vi "Get Topic.vi"(8 "error in (no error)":errorcluster, 9 "Topic Type":variant, 10 "Topic Name":string, 11 "TopicLookupTable in":refnum<class "TopicLookupTable.lvclass">) -> (0 "error out":errorcluster, 1 "Topic Found?":bool, 2 "Topic Refnum":refnum<class "Message Enqueuer.lvclass">, 3 "TopicLookupTable out":refnum<class "TopicLookupTable.lvclass">)   [LabVIEW 2015, in "Mediator.lvlib" / "TopicLookupTable.lvclass"]
uses:
  TopicLookupTable.lvclass
  <vilib>/ActorFramework/Message Enqueuer/Message Enqueuer.lvclass
  TopicLookupTable.lvclass/TopicLookupTable.ctl
  Topic/Topic.lvclass
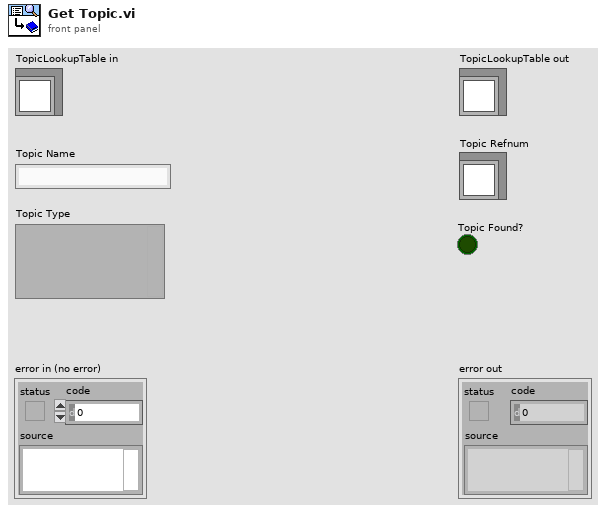
[diagram p1: front panel]
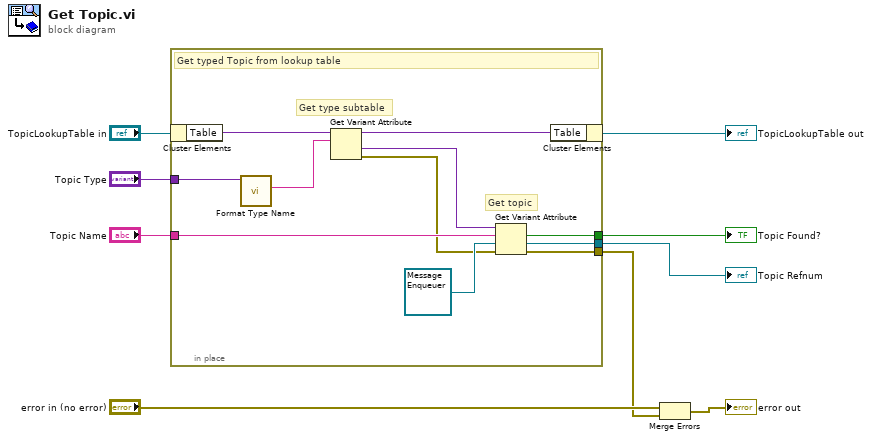
[diagram p0: block diagram]
diagram:
  n1 = in-place {
    in-place-border: "Topic Name" -> [w16]
    in-place-border: "Topic Type" -> [w15]
    in-place-border: [w13] -> w1
    in-place-border: [w12] -> w2
    in-place-border: [w10] -> w3
    # "Get topic"
    # "Get type subtable"
    # "Get typed Topic from lookup table"
    n2 = in-place-cluster #1("TopicLookupTable in") -> ("Table"=w20:variant)
    n3 = call "Format Type Name.vi"("Data Type"=w15) -> ("Name"=w17:string)  [unwired: 9 in, 1 out]
    n4 = Get Variant Attribute(Variant=w20, name=w17) -> (duplicate Variant=w18:variant, value=w19:variant, error out=w11:errorcluster)  [unwired: 2 in, 1 out]
    n5 = Get Variant Attribute(Variant=w19, name=w16, default value (empty Variant)=refnum<class "Message Enqueuer.lvclass"> refnum ("Self Enqueuer"), error in=w11) -> (found=w12:bool, value=w13:refnum<class "Message Enqueuer.lvclass">, error out=w10:errorcluster)  [unwired: 1 out]
    n6 = in-place-cluster #1("Table"=w18) -> (→"TopicLookupTable out":refnum<class "TopicLookupTable.lvclass">)
  }
  "Topic Found?" <- w2
  "Topic Refnum" <- w1
  n7 = Merge Errors("error in (no error)", w3) -> (→"error out":errorcluster)
